vi "KH TURCK ETHERNETIP RFID Init.vi"(8 "err in":errorcluster caption="error", 9 "Timeout":dbl=5.0, 11 "Parameter RFID Array":T1(array[cluster])) -> (0 "err out":errorcluster caption="error")   [LabVIEW 2021]
uses:
  KH TURCK TypeDefs FGlob.ctl
  KH TURCK ETHERNETIP TDef Enum RFID Act Command.ctl
  KH TURCK ETHERNETIP TDef Enum RFID User Command.ctl
  KH TURCK ETHERNETIP RFID Global.vi
  KH TURCK ETHERNETIP Global.vi
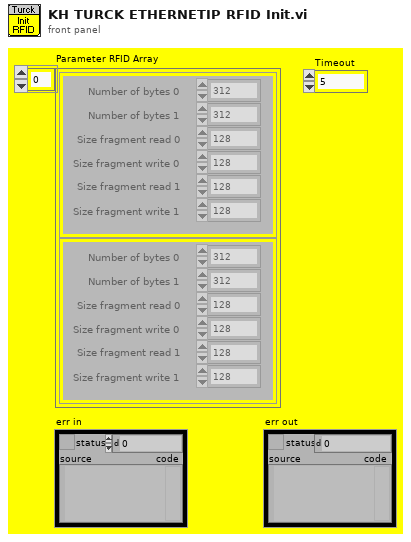
[diagram p1: front panel]
types:
  T1 = cluster{"Number of bytes 0":i32, "SizeFragmentRead1":i32, "SizeFragmentRead0":i32, "SizeFragmentWrite0":i32, "SizeFragmentWrite1":i32, "NumberOfBytes1":i32}[]
  T2 = typedef "KH TURCK TypeDefs FGlob.ctl" = enum16{"Put one", "Put all", "Recall one", "Recall all"}
  T3 = typedef "KH TURCK ETHERNETIP TDefCluster TURCK RFID.ctl" = cluster{"NumberOfBytes":i32, "State":string, "Counter":i32, "ReadData":u8[], "AnzahlFragmente":i32, "WritingFinished":bool, "ReadingFinished":bool, "UID":u8[], "ActCommand":T4, "SizeFragmentRead":i32, "LengthUID":u16, "WriteDataInclUID":u8[], "Timeout":bool, "SizeFragmentWrite":i32}
  T4 = typedef "KH TURCK ETHERNETIP TDef Enum RFID Act Command.ctl" = enum16{"read", "write", "idle", "Inventory", ""}
  T5 = typedef "KH TURCK ETHERNETIP TDef Enum RFID User Command.ctl" = enum16{"read", "write", "idle", "inventory"}
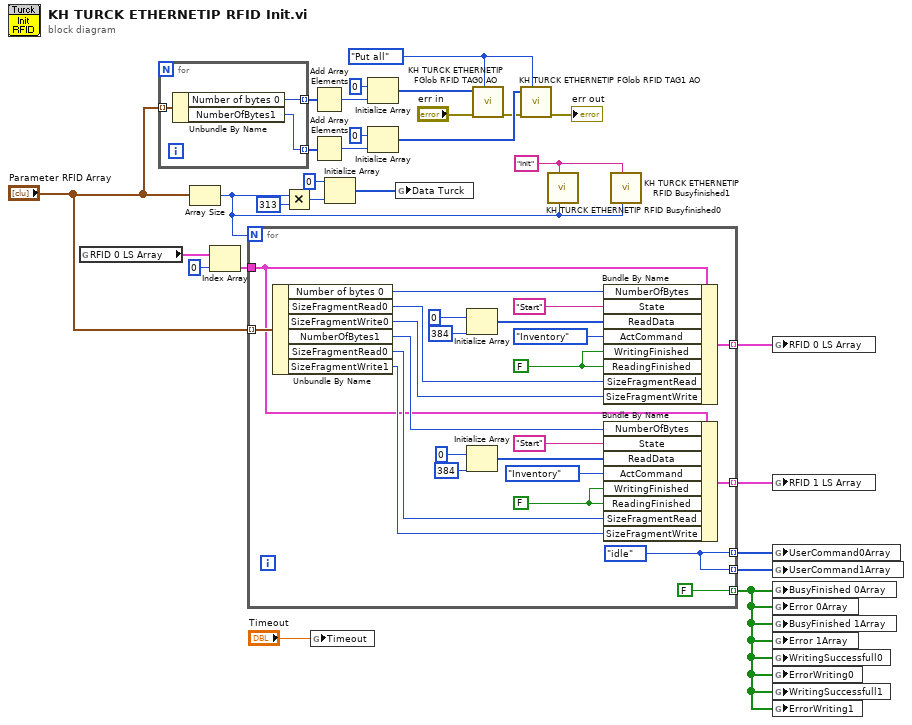
[diagram p0: block diagram]
diagram:
  w16 = KH_TURCK_TypeDefs_FGlob."Put all" ("Function")
  w22 = "Init" ("Function")
  n1 = global read "KH TURCK ETHERNETIP RFID Global.vi" "RFID 0 LS Array"() -> (w24:T3[])
  n2 = for {
    tunnel: "Parameter RFID Array" -> [w31] mode=indexing
    tunnel: [w30] -> w7 mode=indexing
    tunnel: [w29] -> w13 mode=indexing
    n3 = Unbundle By Name(w31) -> ("Number of bytes 0"=w30:i32, "NumberOfBytes1"=w29:i32)
  }
  n4 = Array Size(array="Parameter RFID Array") -> (size(s)=w2:i32)
  n5 = Index Array(array=w24, index=0) -> (element=w23:T3)
  n6 = for {
    N: w2 -> [_]
    tunnel: [w51] -> w28 mode=indexing
    tunnel: [w44] -> w21 mode=indexing
    tunnel: "Parameter RFID Array" -> [w41] mode=indexing
    tunnel: [w32] -> w27 mode=indexing
    tunnel: [w32] -> w26 mode=indexing
    tunnel: w23 -> [w33]
    tunnel: [FALSE ("BusyFinished 0")] -> w5 mode=indexing
    w32 = KH_TURCK_ETHERNETIP_TDef_Enum_RFID_User_Command."idle" ("UserCommand0")
    w48 = FALSE ("WritingFinished")
    w54 = FALSE ("WritingFinished")
    n7 = Unbundle By Name(w41) -> ("Number of bytes 0"=w40:i32, "SizeFragmentRead0"=w39:i32, "SizeFragmentWrite0"=w38:i32, "NumberOfBytes1"=w37:i32, "SizeFragmentRead0"=w36:i32, "SizeFragmentWrite1"=w35:i32)
    n8 = Initialize Array(u8 0 ("Numeric Indicator"), 384 ("dimension size")) -> (w52:u8[])
    n9 = Initialize Array(u8 0 ("Numeric Indicator"), 384 ("dimension size")) -> (w46:u8[])
    n10 = Bundle By Name(cluster=w33, "NumberOfBytes"=w40, "State"="Start", "ReadData"=w52, "ActCommand"=KH_TURCK_ETHERNETIP_TDef_Enum_RFID_Act_Command."Inventory", "WritingFinished"=w54, "ReadingFinished"=w54, "SizeFragmentRead"=w39, "SizeFragmentWrite"=w38) -> (w51:T3)
    n11 = Bundle By Name(cluster=w33, "NumberOfBytes"=w37, "State"="Start", "ReadData"=w46, "ActCommand"=KH_TURCK_ETHERNETIP_TDef_Enum_RFID_Act_Command."Inventory", "WritingFinished"=w48, "ReadingFinished"=w48, "SizeFragmentRead"=w36, "SizeFragmentWrite"=w35) -> (w44:T3)
  }
  n12 = Multiply(x=w2, y=313) -> (x*y=w18:i32)
  n13 = global write "KH TURCK ETHERNETIP RFID Global.vi" "Timeout"("Timeout") -> ()
  n14 = Add Array Elements(numeric array=w7) -> (sum=w8:i32)
  n15 = Add Array Elements(numeric array=w13) -> (sum=w12:i32)
  n16 = Initialize Array(u8 0 ("element"), w18) -> (w1:u8[])
  n17 = Initialize Array(u8 0 ("Numeric"), w8) -> (w14:u8[])
  n18 = Initialize Array(u8 0 ("Numeric"), w12) -> (w15:u8[])
  n19 = global write "KH TURCK ETHERNETIP Global.vi" "Data Turck"(w1) -> ()
  n20 = call "KH TURCK ETHERNETIP FGlob RFID TAG0 AO.vi"("Function"=w16, "err in"="err in", "RFID all in"=w14) -> ("err out"=w9:errorcluster)  [unwired: 6 in, 2 out]
  n21 = call "KH TURCK ETHERNETIP FGlob RFID TAG1 AO.vi"("Function"=w16, "err in"=w9, "RFID all in"=w15) -> ("err out"=→"err out":errorcluster)  [unwired: 6 in, 2 out]
  n22 = call "KH TURCK ETHERNETIP RFID Busyfinished0.vi"("NoOfModules"=w2, "Function"=w22) -> ()  [unwired: 8 in, 2 out]
  n23 = call "KH TURCK ETHERNETIP RFID Busyfinished1.vi"("NoOfModules"=w2, "Function"=w22) -> ()  [unwired: 8 in, 2 out]
  n24 = global write "KH TURCK ETHERNETIP RFID Global.vi" "RFID 0 LS Array"(w28) -> ()
  n25 = global write "KH TURCK ETHERNETIP RFID Global.vi" "RFID 1 LS Array"(w21) -> ()
  n26 = global write "KH TURCK ETHERNETIP RFID Global.vi" "UserCommand0Array"(w26) -> ()
  n27 = global write "KH TURCK ETHERNETIP RFID Global.vi" "UserCommand1Array"(w27) -> ()
  n28 = global write "KH TURCK ETHERNETIP RFID Global.vi" "BusyFinished 0Array"(w5) -> ()
  n29 = global write "KH TURCK ETHERNETIP RFID Global.vi" "Error 0Array"(w5) -> ()
  n30 = global write "KH TURCK ETHERNETIP RFID Global.vi" "BusyFinished 1Array"(w5) -> ()
  n31 = global write "KH TURCK ETHERNETIP RFID Global.vi" "Error 1Array"(w5) -> ()
  n32 = global write "KH TURCK ETHERNETIP RFID Global.vi" "WritingSuccessfull0"(w5) -> ()
  n33 = global write "KH TURCK ETHERNETIP RFID Global.vi" "ErrorWriting0"(w5) -> ()
  n34 = global write "KH TURCK ETHERNETIP RFID Global.vi" "WritingSuccessfull1"(w5) -> ()
  n35 = global write "KH TURCK ETHERNETIP RFID Global.vi" "ErrorWriting1"(w5) -> ()
